vi "simx Get Joint Matrix.vi"(7 "operationMode":i32, 8 "error in (no error)":errorcluster, 9 "matrix":sgl, 10 "jointHandle":i32, 11 "clientID":i32) -> (0 "error out":errorcluster, 1 "matrix out":sgl, 3 "function return":i32)   [LabVIEW 2019, in "PXL_V-REP.lvlib"]
doc: "EXTAPI_DLLEXPORT simxInt simxGetJointMatrix(simxInt clientID,simxInt jointHandle,simxFloat* matrix,simxInt operationMode);"
uses:
  PXL_V-REP.lvlib
  <userlib>/V-REP/remoteApi.dll
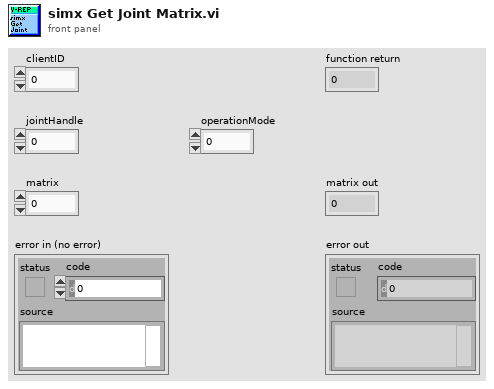
[diagram p1: front panel]
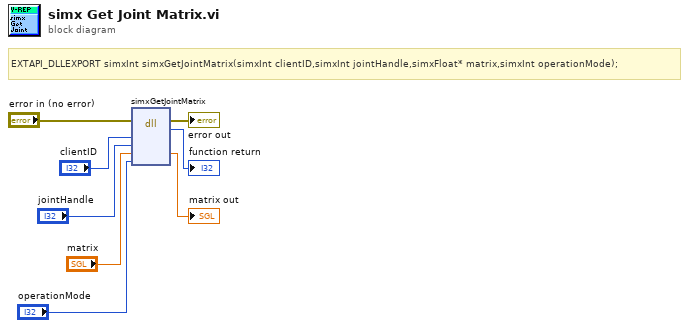
[diagram p0: block diagram]
diagram:
  # "EXTAPI_DLLEXPORT simxInt simxGetJointMatrix(simxInt clientID,simxInt jointHandle,simxFloat* matrix,simxInt operationMode);"
  n1 = dll-call lib="C:/Program Files (x86)/National Instruments/LabVIEW 2019/user.lib/V-REP/remoteApi.*" fn="simxGetJointMatrix"(error in="error in (no error)", "clientID"="clientID", "jointHandle"="jointHandle", "matrix"="matrix", "operationMode"="operationMode") -> (error out=→"error out":errorcluster, →"function return":i32, "matrix"=→"matrix out":sgl)  [unwired: 5 in, 1 out]
